vi "总磷总氮测量数据储存.vi"   [LabVIEW 2016, in "斯坦道CODcr.lvlib"]
types:
  T1 = enum16{"水样测试", "标样核查", "跨度核查", "零点核查", "加标回收", "空白测试", "平行样"}
  T2 = cluster{"时间标识":timestamp, "测量模式":enum16{"维护数据", "水样测试", "标样核查", "零点核查", "跨度核查", "空白测试", "平行样测试", "加标回收", "空白校准", "标样校准", "初始化（清洗）", "快捷测试"}, "数据标记表":string, "监测值":sgl, "单位":u16, "数据标识":string, "因子编码":u32, "标样参考值":sgl, "F0":sgl, "F1":sgl, "F2":sgl, "F3":sgl, "F4":sgl, "F5":sgl, "F6":sgl, "F7":sgl, "X":sgl, "温度":sgl, "湿度":sgl, "量程标识":string, "SN":string, "跨度值":sgl, "X1":sgl}
  T3 = enum16{"维护数据", "水样测试", "标样核查", "零点核查", "跨度核查", "空白测试", "平行样测试", "加标回收", "空白校准", "标样校准", "初始化（清洗）", "快捷测试"}
  T4 = enum16{"维护数据", "水样测试", "标样核查", "零点核查", "跨度核查", "空白测试", "平行样测试", "加标回收", "空白校准", "标样校准", "初始化（清洗）"}
  T5 = cluster{"系统时间":timestamp, "工作状态":u16, "测量模式":enum16{"待机", "连续模式", "周期模式", "定点模式", "受控模式", "手动模式"}, "告警代码":u16, "故障代码":u16, "日志代码":u16, "软件版本":u16, "F0":sgl, "F1":sgl, "F2":sgl, "F3":sgl, "T":sgl, "H":sgl, "id":u16, "flowid":u16, "量程":u16, "总磷控温温度1":sgl, "营养盐控温温度2":sgl, "ADC":sgl}
  T6 = cluster{"运行模式":enum16{"维护模式", "常规模式", "应急模式", "质控模式"}, "质控频次":enum16{"关闭", "每天", "星期一", "星期二", "星期三", "星期四", "星期五", "星期六", "星期日"}, "空白核查时间":u16, "跨度核查时间":u16, "测量间隔":u16}
  T7 = cluster{"因子编码":u32, "单位":u16, "标样参考值":sgl, "水样数据时间":timestamp, "水样实测值":sgl, "水样数据标识":string, "标样数据时间":timestamp, "标样实测值":sgl, "标样数据标识":string, "空白数据时间":timestamp, "空白实测值":sgl, "空白数据标识":string, "零点核查数据时间":timestamp, "零点核查实测值":sgl, "零点核查数据标识":string, "跨度核查数据时间":timestamp, "跨度核查实测值":sgl, "跨度核查数据标识":string, "加标回收数据时间":timestamp, "加标回收实测值":sgl, "加标回收数据标识":string, "平行样数据时间":timestamp, "平行样实测值":sgl, "平行样数据标识":string, "F0":sgl, "F1":sgl, "F2":sgl, "F3":sgl, "F4":sgl, "F5":sgl, "F6":sgl, "F7":sgl, "温度":sgl, "湿度":sgl, "X值":sgl, "fidrange":u16, "X1值":sgl}[]
  T8 = cluster{"因子编码":u32, "单位":u16, "标样参考值":sgl, "水样数据时间":timestamp, "水样实测值":sgl, "水样数据标识":string, "标样数据时间":timestamp, "标样实测值":sgl, "标样数据标识":string, "空白数据时间":timestamp, "空白实测值":sgl, "空白数据标识":string, "零点核查数据时间":timestamp, "零点核查实测值":sgl, "零点核查数据标识":string, "跨度核查数据时间":timestamp, "跨度核查实测值":sgl, "跨度核查数据标识":string, "加标回收数据时间":timestamp, "加标回收实测值":sgl, "加标回收数据标识":string, "平行样数据时间":timestamp, "平行样实测值":sgl, "平行样数据标识":string, "F0":sgl, "F1":sgl, "F2":sgl, "F3":sgl, "F4":sgl, "F5":sgl, "F6":sgl, "F7":sgl, "温度":sgl, "湿度":sgl, "X值":sgl, "fidrange":u16, "X1值":sgl}
  T9 = cluster{"总磷跨度值":dbl, "总磷零点标准液浓度":dbl, "总磷跨度标准液浓度":dbl, "总磷标准液标准浓度":dbl, "总氮跨度值":dbl, "总氮零点标准液浓度":dbl, "总氮跨度标准液浓度":dbl, "总氮标准液标准浓度":dbl, "COD跨度值":dbl, "COD零点标准液浓度":dbl, "COD跨度标准液浓度":dbl, "COD标准液标准浓度":dbl, "氨氮跨度值":dbl, "氨氮零点标准液浓度":dbl, "氨氮跨度标准液浓度":dbl, "氨氮标准液标准浓度":dbl, "磷酸盐跨度值":dbl, "磷酸盐零点标准液浓度":dbl, "磷酸盐跨度标准液浓度":dbl, "磷酸盐标准液标准浓度":dbl, "硝氮跨度值":dbl, "硝氮零点标准液浓度":dbl, "硝氮跨度标准液浓度":dbl, "硝氮标准液标准浓度":dbl, "亚硝氮跨度值":dbl, "亚硝氮零点标准液浓度":dbl, "亚硝氮跨度标准液浓度":dbl, "亚硝氮标准液标准浓度":dbl, "硫化物跨度值":dbl, "硫化物零点标准液浓度":dbl, "硫化物跨度标准液浓度":dbl, "硫化物标准液标准浓度":dbl, "硅酸盐跨度值":dbl, "硅酸盐零点标准液浓度":dbl, "硅酸盐跨度标准液浓度":dbl, "硅酸盐标准液标准浓度":dbl}
  T10 = typedef "斯坦道CODcr.lvlib/关键参数.ctl" = cluster{"测量量程":sgl, "测量检出限":sgl, "测量精度":sgl, "测量间隔":sgl, "消解温度":sgl, "消解时长":sgl, "三项式系数":sgl, "二次多项式系数":sgl, "曲线斜率":sgl, "曲线截距":sgl, "线性相关系数":sgl, "空白校准时间":timestamp, "标样校准时间":timestamp, "测量信号值":sgl, "稀释倍数":sgl, "空白标定系数":sgl, "量程系数":sgl}
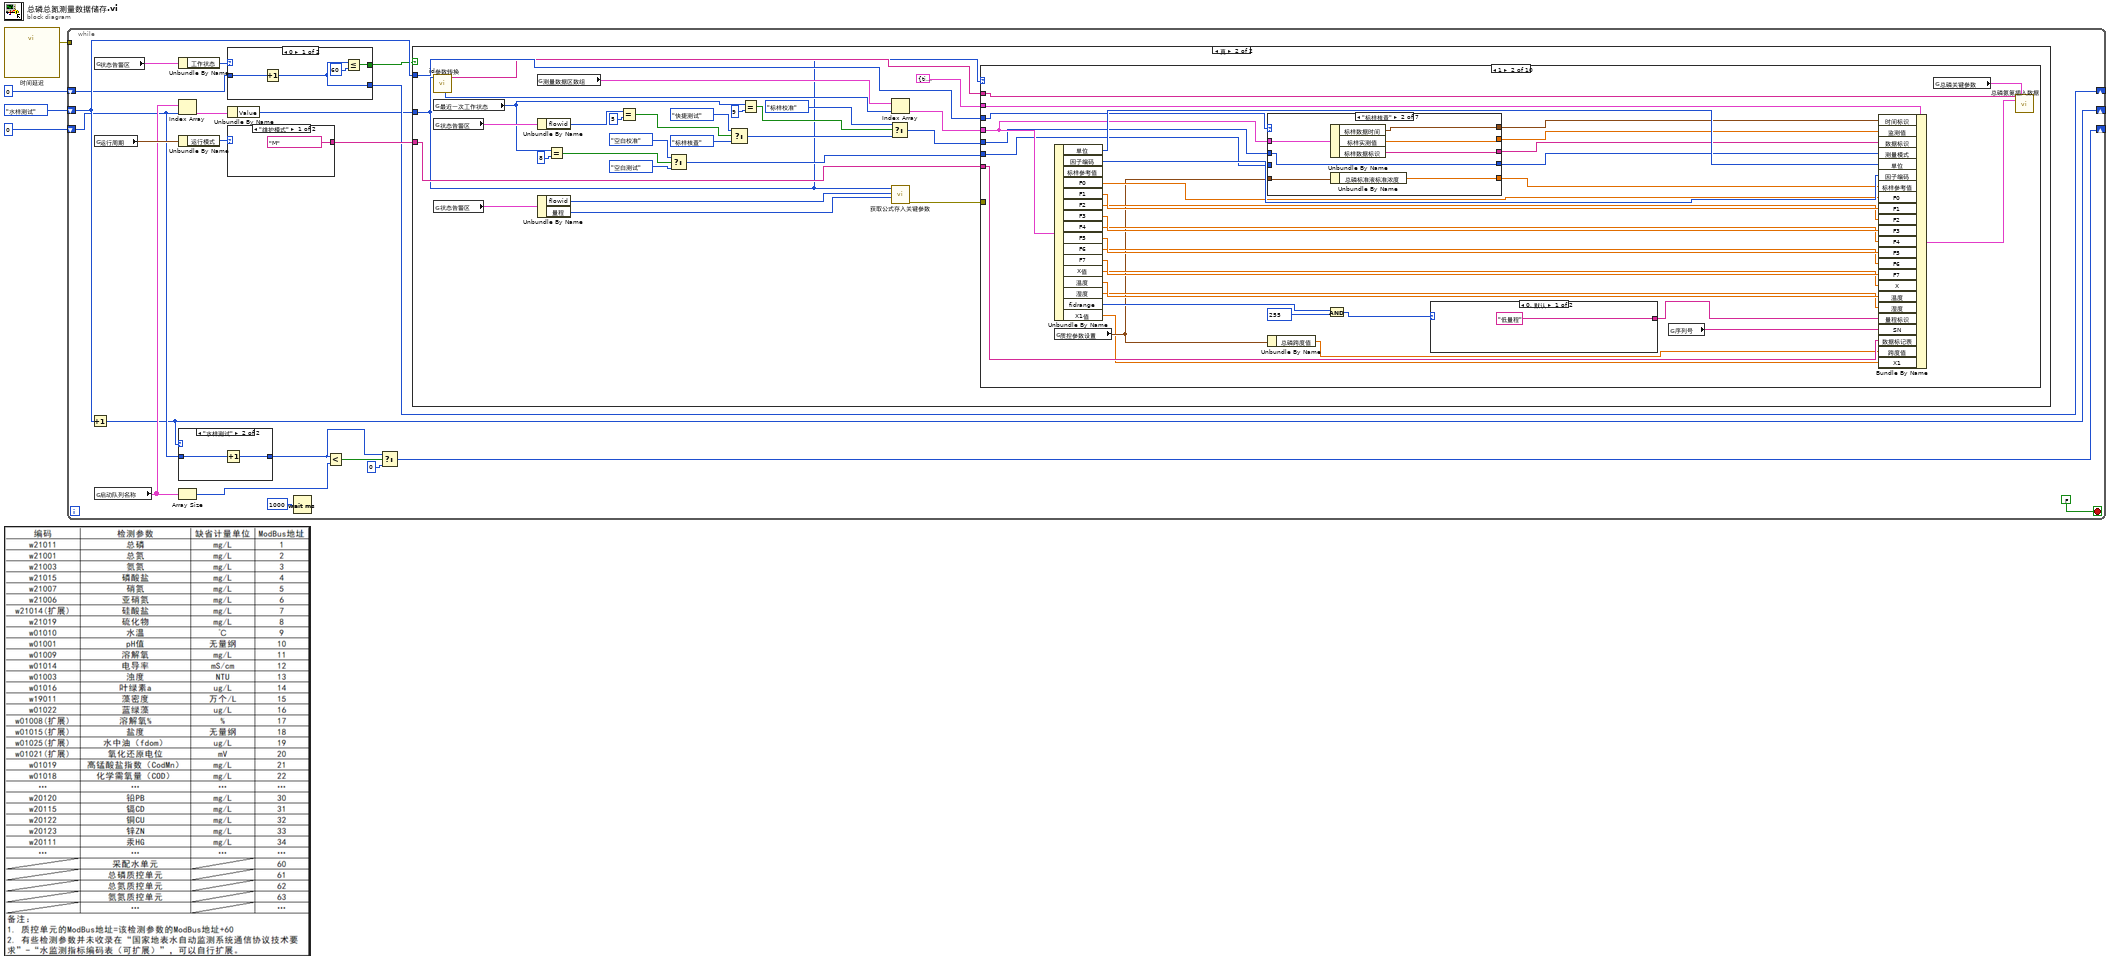
[diagram p0: block diagram]
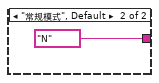
[diagram p4: hidden frame]
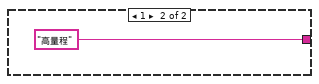
[diagram p7: hidden frame]
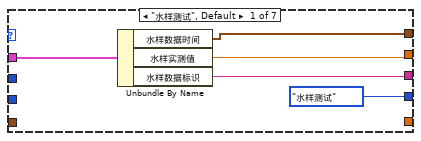
[diagram p8: hidden frame]
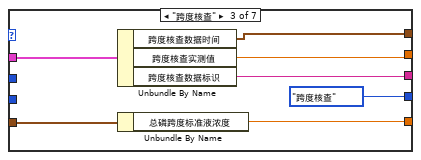
[diagram p9: hidden frame]
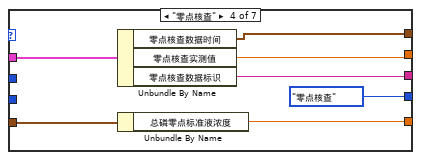
[diagram p10: hidden frame]
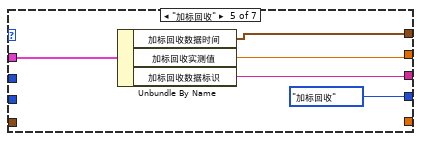
[diagram p11: hidden frame]
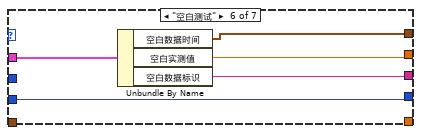
[diagram p12: hidden frame]
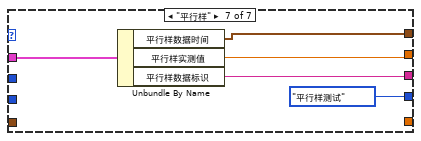
[diagram p13: hidden frame]
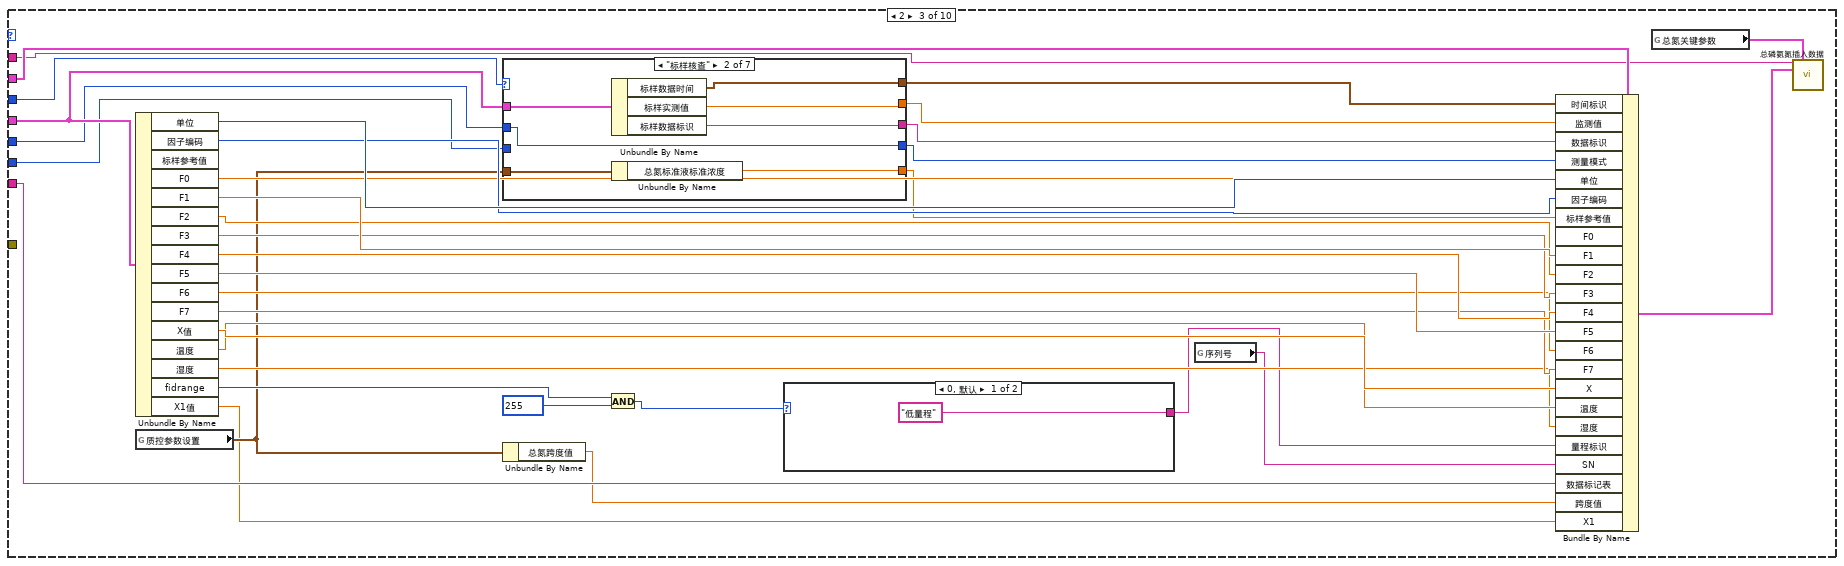
[diagram p14: hidden frame]
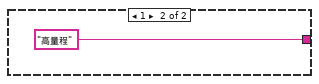
[diagram p15: hidden frame]
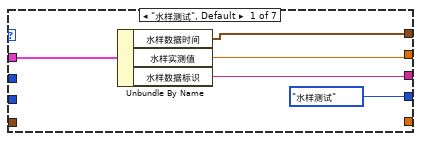
[diagram p16: hidden frame]
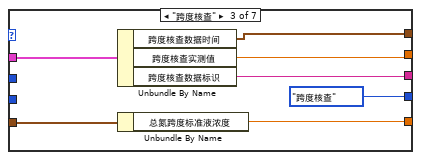
[diagram p17: hidden frame]
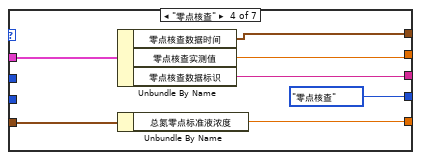
[diagram p18: hidden frame]
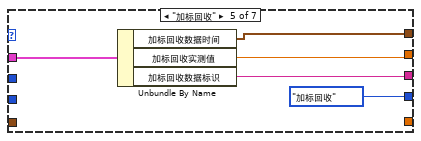
[diagram p19: hidden frame]
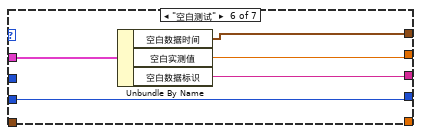
[diagram p20: hidden frame]
diagram:
  n1 = call "时间延迟"() -> ("error out"=w2:errorcluster)  [unwired: 11 in]
  n2 = while {
    shift-right: [w7] -> _
    shift-left: T1."水样测试" ("测量模式") -> [w23]
    shift-right: [w17] -> _
    shift-left: u32 0 ("等待时间（毫秒）") -> [w18]
    tunnel: w2 -> [_]
    shift-right: [w8] -> _
    shift-left: 0 -> [w11]
    stop <- FALSE stop-if-true
    n3 = Increment(x=w23) -> (x+1=w7:T1)
    n4 = global read "VAR总磷总氮全局变量.vi" "状态告警区"() -> (w20:T5)
    n5 = global read "总磷总氮断电保存全局变量.vi" "运行周期"() -> (w22:T6)
    n6 = global read "model config var.vi" "启动队列名称"() -> (w12:cluster{"String":string, "Value":u16}[])
    n7 = Unbundle By Name(w20) -> ("工作状态"=w19:u16)
    n8 = Index Array(array=w12, index=w11) -> (element=w14:cluster{"String":string, "Value":u16})
    n9 = Unbundle By Name(w22) -> ("运行模式"=w21:enum16{"维护模式", "常规模式", "应急模式", "质控模式"})
    n10 = case shown="\"水样测试\"" w7 {
      tunnel: w11 -> [w26 w28]
      tunnel: [w26 w27] -> w5
      frame Default {
      }
      frame "水样测试" {
        n11 = Increment(x=w28) -> (x+1=w27:i32)
      }
    }
    n12 = Array Size(array=w12) -> (size(s)=w10:i32)
    n13 = case shown="0" w19 {
      tunnel: w18 -> [w32 _]
      tunnel: [w31 _] -> w17
      tunnel: [w29 _] -> w16
      frame 0 {
        n14 = Increment(x=w32) -> (x+1=w31:u32)
        n15 = Less Or Equal?(x=w31, y=u32 60) -> (x <= y?=w29:bool)
      }
      frame 1, Default {
      }
    }
    n16 = Unbundle By Name(w14) -> ("Value"=w13:u16)
    n17 = case shown="\"维护模式\"" w21 {
      tunnel: ["M" ("数据标记表") "N" ("数据标记表")] -> w24
      frame "维护模式" {
      }
      frame "常规模式", Default {
      }
    }
    n18 = Wait (ms)(milliseconds to wait=u32 1000 ("等待时间（毫秒）")) -> ()  [unwired: 1 out]
    n19 = Less?(x=w5, y=w10) -> (x < y?=w9:bool)
    n20 = Select(t=w5, s=w9, f=0) -> (s? t:f=w8:i32)
    n21 = case shown="真" w16 {
      tunnel: w24 -> [_ w63]
      tunnel: w23 -> [_ w62]
      tunnel: w13 -> [_ w35]
      frame False {
      }
      frame True {
        n22 = call "id参数转换.vi"("id"=w35) -> ("table输出"=w58:string, "数组资源索引"=w57:i32)  [unwired: 9 in]
        n23 = global read "VAR总磷总氮全局变量.vi" "最近一次工作状态"() -> (w49:u16)
        n24 = global read "VAR总磷总氮全局变量.vi" "状态告警区"() -> (w61:T5)
        n25 = global read "VAR总磷总氮全局变量.vi" "状态告警区"() -> (w39:T5)
        n26 = global read "VAR总磷总氮全局变量.vi" "测量数据区数组"() -> (w60:T7)
        n27 = Unbundle By Name(w61) -> ("flowid"=w46:u16)
        n28 = Unbundle By Name(w39) -> ("flowid"=w38:u16, "量程"=w37:u16)
        n29 = Equal?(x=w49, y=u16 8) -> (x = y?=w55:bool)
        n30 = Equal?(x=w46, y=u16 5) -> (x = y?=w44:bool)
        n31 = Select(t=T3."空白校准" ("测量模式"), s=w55, f=T3."空白测试" ("测量模式")) -> (s? t:f=w48:T3)
        n32 = Select(t=T3."快捷测试" ("测量模式"), s=w44, f=T3."标样核查" ("测量模式")) -> (s? t:f=w41:T3)
        n33 = Equal?(x=w49, y=u16 9) -> (x = y?=w51:bool)
        n34 = Select(t=T3."标样校准" ("测量模式"), s=w51, f=w41) -> (s? t:f=w47:T3)
        n35 = Index Array(array=w60, index=w57) -> (element=w59:T8)
        n36 = call "获取公式存入关键参数.vi"("量程"=w37, "flowid"=w38, "id"=w35) -> ("error out"=w36:errorcluster)  [unwired: 8 in]
        n37 = case shown="1" w35 {
          tunnel: w63 -> [_ w74 w152 w231 w309 w387 w465 w543 w621 w699]
          tunnel: w62 -> [_ w82 w163 w241 w319 w397 w475 w553 w631 w709]
          tunnel: T2 {"时间标识"=timestamp(0 s since 1904-01-01), "测量模式"=enum."水样测试", "数据标记表"="N", "监测值"=0.0, "单位"=0, "数据标识"="", "因子编码"=0, "标样参考值"=0.0, "F0"=0.0, "F1"=0.0, "F2"=0.0, "F3"=0.0, "F4"=0.0, "F5"=0.0, "F6"=0.0, "F7"=0.0, "X"=0.0, "温度"=0.0, "湿度"=0.0, "量程标识"="", "SN"="", "跨度值"=0.0, "X1"=0.0} ("data") -> [_ w72 w150 w229 w307 w385 w463 w541 w619 w697]
          tunnel: w59 -> [_ w69 w147 w226 w304 w382 w460 w538 w616 w693]
          tunnel: w58 -> [_ w68 w146 w224 w302 w380 w458 w536 w614 w692]
          tunnel: w48 -> [_ w67 w145 w222 w301 w379 w457 w534 w613 w691]
          tunnel: w47 -> [_ w66 w144 w223 w300 w378 w456 w535 w612 w690]
          tunnel: w36 -> [_ _ _ _ _ _ _ _ _ _]
          frame Default {
          }
          frame 1 {
            n38 = Unbundle By Name(w69) -> ("单位"=w98:u16, "因子编码"=w97:u32, "F0"=w96:sgl, "F1"=w95:sgl, "F2"=w94:sgl, "F3"=w93:sgl, "F4"=w92:sgl, "F5"=w91:sgl, "F6"=w90:sgl, "F7"=w89:sgl, "X值"=w88:sgl, "温度"=w87:sgl, "湿度"=w86:sgl, "fidrange"=w80:u16, "X1值"=w64:sgl)  [unwired: 1 out]
            n39 = global read "总磷总氮断电保存全局变量.vi" "质控参数设置"() -> (w71:T9)
            n40 = case shown="\"标样核查\"" w82 {
              tunnel: w69 -> [w105 w112 w119 w126 w131 w136 w141]
              tunnel: [w104 w111 w118 w125 w130 w135 w140] -> w83
              tunnel: [w103 w110 w117 w124 w129 w134 w139] -> w84
              tunnel: [w102 w109 w116 w123 w128 w133 w138] -> w85
              tunnel: [T4."水样测试" ("测量模式") w106 T4."跨度核查" ("测量模式") T4."零点核查" ("测量模式") T4."加标回收" ("测量模式") w132 T4."平行样测试" ("测量模式")] -> w73
              tunnel: w71 -> [_ w108 w114 w121 _ _ _]
              tunnel: [_ w107 w113 w120 _ _ _] -> w81
              tunnel: w67 -> [_ _ _ _ _ w132 _]
              tunnel: w66 -> [_ w106 _ _ _ _ _]
              frame "水样测试", Default {
                n41 = Unbundle By Name(w105) -> ("水样数据时间"=w104:timestamp, "水样实测值"=w103:sgl, "水样数据标识"=w102:string)
              }
              frame "标样核查" {
                n42 = Unbundle By Name(w112) -> ("标样数据时间"=w111:timestamp, "标样实测值"=w110:sgl, "标样数据标识"=w109:string)
                n43 = Unbundle By Name(w108) -> ("总磷标准液标准浓度"=w107:dbl)
              }
              frame "跨度核查" {
                n44 = Unbundle By Name(w119) -> ("跨度核查数据时间"=w118:timestamp, "跨度核查实测值"=w117:sgl, "跨度核查数据标识"=w116:string)
                n45 = Unbundle By Name(w114) -> ("总磷跨度标准液浓度"=w113:dbl)
              }
              frame "零点核查" {
                n46 = Unbundle By Name(w126) -> ("零点核查数据时间"=w125:timestamp, "零点核查实测值"=w124:sgl, "零点核查数据标识"=w123:string)
                n47 = Unbundle By Name(w121) -> ("总磷零点标准液浓度"=w120:dbl)
              }
              frame "加标回收" {
                n48 = Unbundle By Name(w131) -> ("加标回收数据时间"=w130:timestamp, "加标回收实测值"=w129:sgl, "加标回收数据标识"=w128:string)
              }
              frame "空白测试" {
                n49 = Unbundle By Name(w136) -> ("空白数据时间"=w135:timestamp, "空白实测值"=w134:sgl, "空白数据标识"=w133:string)
              }
              frame "平行样" {
                n50 = Unbundle By Name(w141) -> ("平行样数据时间"=w140:timestamp, "平行样实测值"=w139:sgl, "平行样数据标识"=w138:string)
              }
            }
            n51 = Unbundle By Name(w71) -> ("总磷跨度值"=w70:dbl)
            n52 = And(x=w80, y=u16 255) -> (x .and. y?=w78:u16)
            n53 = case shown="0, 默认" w78 {
              tunnel: ["低量程" ("格式字符串") "高量程" ("格式字符串")] -> w77
              frame 0, Default {
              }
              frame 1 {
              }
            }
            n54 = global read "VAR总磷总氮全局变量.vi" "序列号"() -> (w75:string)
            n55 = Bundle By Name(cluster=w72, "时间标识"=w83, "监测值"=w84, "数据标识"=w85, "测量模式"=w73, "单位"=w98, "因子编码"=w97, "标样参考值"=w81, "F0"=w96, "F1"=w95, "F2"=w94, "F3"=w93, "F4"=w92, "F5"=w91, "F6"=w90, "F7"=w89, "X"=w88, "温度"=w87, "湿度"=w86, "量程标识"=w77, "SN"=w75, "数据标记表"=w74, "跨度值"=w70, "X1"=w64) -> (w76:T2)
            n56 = global read "VAR总磷总氮全局变量.vi" "总磷关键参数"() -> (w65:T10)
            n57 = call "总磷氨氮插入数据.vi"("table"=w68, "关键参数"=w65, "data"=w76) -> ()  [unwired: 12 in, 1 out]
          }
          frame 2 {
            n58 = Unbundle By Name(w147) -> ("单位"=w176:u16, "因子编码"=w175:u32, "F0"=w174:sgl, "F1"=w173:sgl, "F2"=w172:sgl, "F3"=w171:sgl, "F4"=w170:sgl, "F5"=w169:sgl, "F6"=w168:sgl, "F7"=w167:sgl, "X值"=w166:sgl, "温度"=w165:sgl, "湿度"=w164:sgl, "fidrange"=w156:u16, "X1值"=w142:sgl)  [unwired: 1 out]
            n59 = global read "总磷总氮断电保存全局变量.vi" "质控参数设置"() -> (w149:T9)
            n60 = case shown="\"标样核查\"" w163 {
              tunnel: w147 -> [w183 w190 w197 w204 w209 w214 w219]
              tunnel: [w182 w189 w196 w203 w208 w213 w218] -> w162
              tunnel: [w181 w188 w195 w202 w207 w212 w217] -> w161
              tunnel: [w180 w187 w194 w201 w206 w211 w216] -> w160
              tunnel: [T4."水样测试" ("测量模式") w184 T4."跨度核查" ("测量模式") T4."零点核查" ("测量模式") T4."加标回收" ("测量模式") w210 T4."平行样测试" ("测量模式")] -> w151
              tunnel: w149 -> [_ w186 w192 w199 _ _ _]
              tunnel: [_ w185 w191 w198 _ _ _] -> w159
              tunnel: w145 -> [_ _ _ _ _ w210 _]
              tunnel: w144 -> [_ w184 _ _ _ _ _]
              frame "水样测试", Default {
                n61 = Unbundle By Name(w183) -> ("水样数据时间"=w182:timestamp, "水样实测值"=w181:sgl, "水样数据标识"=w180:string)
              }
              frame "标样核查" {
                n62 = Unbundle By Name(w190) -> ("标样数据时间"=w189:timestamp, "标样实测值"=w188:sgl, "标样数据标识"=w187:string)
                n63 = Unbundle By Name(w186) -> ("总氮标准液标准浓度"=w185:dbl)
              }
              frame "跨度核查" {
                n64 = Unbundle By Name(w197) -> ("跨度核查数据时间"=w196:timestamp, "跨度核查实测值"=w195:sgl, "跨度核查数据标识"=w194:string)
                n65 = Unbundle By Name(w192) -> ("总氮跨度标准液浓度"=w191:dbl)
              }
              frame "零点核查" {
                n66 = Unbundle By Name(w204) -> ("零点核查数据时间"=w203:timestamp, "零点核查实测值"=w202:sgl, "零点核查数据标识"=w201:string)
                n67 = Unbundle By Name(w199) -> ("总氮零点标准液浓度"=w198:dbl)
              }
              frame "加标回收" {
                n68 = Unbundle By Name(w209) -> ("加标回收数据时间"=w208:timestamp, "加标回收实测值"=w207:sgl, "加标回收数据标识"=w206:string)
              }
              frame "空白测试" {
                n69 = Unbundle By Name(w214) -> ("空白数据时间"=w213:timestamp, "空白实测值"=w212:sgl, "空白数据标识"=w211:string)
              }
              frame "平行样" {
                n70 = Unbundle By Name(w219) -> ("平行样数据时间"=w218:timestamp, "平行样实测值"=w217:sgl, "平行样数据标识"=w216:string)
              }
            }
            n71 = Unbundle By Name(w149) -> ("总氮跨度值"=w148:dbl)
            n72 = And(x=w156, y=u16 255) -> (x .and. y?=w157:u16)
            n73 = case shown="0, 默认" w157 {
              tunnel: ["低量程" ("格式字符串") "高量程" ("格式字符串")] -> w155
              frame 0, Default {
              }
              frame 1 {
              }
            }
            n74 = global read "VAR总磷总氮全局变量.vi" "序列号"() -> (w153:string)
            n75 = Bundle By Name(cluster=w150, "时间标识"=w162, "监测值"=w161, "数据标识"=w160, "测量模式"=w151, "单位"=w176, "因子编码"=w175, "标样参考值"=w159, "F0"=w174, "F1"=w173, "F2"=w172, "F3"=w171, "F4"=w170, "F5"=w169, "F6"=w168, "F7"=w167, "X"=w166, "温度"=w165, "湿度"=w164, "量程标识"=w155, "SN"=w153, "数据标记表"=w152, "跨度值"=w148, "X1"=w142) -> (w154:T2)
            n76 = global read "VAR总磷总氮全局变量.vi" "总氮关键参数"() -> (w143:T10)
            n77 = call "总磷氨氮插入数据.vi"("table"=w146, "关键参数"=w143, "data"=w154) -> ()  [unwired: 12 in, 1 out]
          }
          frame 3 {
            n78 = Unbundle By Name(w226) -> ("单位"=w254:u16, "因子编码"=w253:u32, "F0"=w252:sgl, "F1"=w251:sgl, "F2"=w250:sgl, "F3"=w249:sgl, "F4"=w248:sgl, "F5"=w247:sgl, "F6"=w246:sgl, "F7"=w245:sgl, "X值"=w244:sgl, "温度"=w243:sgl, "湿度"=w242:sgl, "fidrange"=w234:u16, "X1值"=w220:sgl)  [unwired: 1 out]
            n79 = global read "总磷总氮断电保存全局变量.vi" "质控参数设置"() -> (w228:T9)
            n80 = case shown="\"空白测试\"" w241 {
              tunnel: w226 -> [w261 w268 w275 w282 w287 w292 w297]
              tunnel: [w260 w267 w274 w281 w286 w291 w296] -> w240
              tunnel: [w259 w266 w273 w280 w285 w290 w295] -> w239
              tunnel: [w258 w265 w272 w279 w284 w289 w294] -> w238
              tunnel: [T4."水样测试" ("测量模式") w262 T4."跨度核查" ("测量模式") T4."零点核查" ("测量模式") T4."加标回收" ("测量模式") w288 T4."平行样测试" ("测量模式")] -> w230
              tunnel: w228 -> [_ w264 w270 w277 _ _ _]
              tunnel: [_ w263 w269 w276 _ _ _] -> w237
              tunnel: w223 -> [_ w262 _ _ _ _ _]
              tunnel: w222 -> [_ _ _ _ _ w288 _]
              frame "水样测试", Default {
                n81 = Unbundle By Name(w261) -> ("水样数据时间"=w260:timestamp, "水样实测值"=w259:sgl, "水样数据标识"=w258:string)
              }
              frame "标样核查" {
                n82 = Unbundle By Name(w268) -> ("标样数据时间"=w267:timestamp, "标样实测值"=w266:sgl, "标样数据标识"=w265:string)
                n83 = Unbundle By Name(w264) -> ("氨氮标准液标准浓度"=w263:dbl)
              }
              frame "跨度核查" {
                n84 = Unbundle By Name(w275) -> ("跨度核查数据时间"=w274:timestamp, "跨度核查实测值"=w273:sgl, "跨度核查数据标识"=w272:string)
                n85 = Unbundle By Name(w270) -> ("氨氮跨度标准液浓度"=w269:dbl)
              }
              frame "零点核查" {
                n86 = Unbundle By Name(w282) -> ("零点核查数据时间"=w281:timestamp, "零点核查实测值"=w280:sgl, "零点核查数据标识"=w279:string)
                n87 = Unbundle By Name(w277) -> ("氨氮零点标准液浓度"=w276:dbl)
              }
              frame "加标回收" {
                n88 = Unbundle By Name(w287) -> ("加标回收数据时间"=w286:timestamp, "加标回收实测值"=w285:sgl, "加标回收数据标识"=w284:string)
              }
              frame "空白测试" {
                n89 = Unbundle By Name(w292) -> ("空白数据时间"=w291:timestamp, "空白实测值"=w290:sgl, "空白数据标识"=w289:string)
              }
              frame "平行样" {
                n90 = Unbundle By Name(w297) -> ("平行样数据时间"=w296:timestamp, "平行样实测值"=w295:sgl, "平行样数据标识"=w294:string)
              }
            }
            n91 = Unbundle By Name(w228) -> ("氨氮跨度值"=w227:dbl)
            n92 = And(x=w234, y=u16 255) -> (x .and. y?=w235:u16)
            n93 = case shown="0, 默认" w235 {
              tunnel: ["低量程" ("格式字符串") "高量程" ("格式字符串")] -> w233
              frame 0, Default {
              }
              frame 1 {
              }
            }
            n94 = global read "VAR总磷总氮全局变量.vi" "序列号"() -> (w232:string)
            n95 = Bundle By Name(cluster=w229, "时间标识"=w240, "监测值"=w239, "数据标识"=w238, "测量模式"=w230, "单位"=w254, "因子编码"=w253, "标样参考值"=w237, "F0"=w252, "F1"=w251, "F2"=w250, "F3"=w249, "F4"=w248, "F5"=w247, "F6"=w246, "F7"=w245, "X"=w244, "温度"=w243, "湿度"=w242, "量程标识"=w233, "SN"=w232, "数据标记表"=w231, "跨度值"=w227, "X1"=w220) -> (w225:T2)
            n96 = global read "VAR总磷总氮全局变量.vi" "氨氮关键参数"() -> (w221:T10)
            n97 = call "总磷氨氮插入数据.vi"("table"=w224, "关键参数"=w221, "data"=w225) -> ()  [unwired: 12 in, 1 out]
          }
          frame 4 {
            n98 = Unbundle By Name(w304) -> ("单位"=w332:u16, "因子编码"=w331:u32, "F0"=w330:sgl, "F1"=w329:sgl, "F2"=w328:sgl, "F3"=w327:sgl, "F4"=w326:sgl, "F5"=w325:sgl, "F6"=w324:sgl, "F7"=w323:sgl, "X值"=w322:sgl, "温度"=w321:sgl, "湿度"=w320:sgl, "fidrange"=w312:u16, "X1值"=w298:sgl)  [unwired: 1 out]
            n99 = global read "总磷总氮断电保存全局变量.vi" "质控参数设置"() -> (w306:T9)
            n100 = case shown="\"标样核查\"" w319 {
              tunnel: w304 -> [w339 w346 w353 w360 w365 w370 w375]
              tunnel: [w338 w345 w352 w359 w364 w369 w374] -> w318
              tunnel: [w337 w344 w351 w358 w363 w368 w373] -> w317
              tunnel: [w336 w343 w350 w357 w362 w367 w372] -> w316
              tunnel: [T4."水样测试" ("测量模式") w340 T4."跨度核查" ("测量模式") T4."零点核查" ("测量模式") T4."加标回收" ("测量模式") w366 T4."平行样测试" ("测量模式")] -> w308
              tunnel: w306 -> [_ w342 w348 w355 _ _ _]
              tunnel: [_ w341 w347 w354 _ _ _] -> w315
              tunnel: w301 -> [_ _ _ _ _ w366 _]
              tunnel: w300 -> [_ w340 _ _ _ _ _]
              frame "水样测试", Default {
                n101 = Unbundle By Name(w339) -> ("水样数据时间"=w338:timestamp, "水样实测值"=w337:sgl, "水样数据标识"=w336:string)
              }
              frame "标样核查" {
                n102 = Unbundle By Name(w346) -> ("标样数据时间"=w345:timestamp, "标样实测值"=w344:sgl, "标样数据标识"=w343:string)
                n103 = Unbundle By Name(w342) -> ("磷酸盐标准液标准浓度"=w341:dbl)
              }
              frame "跨度核查" {
                n104 = Unbundle By Name(w353) -> ("跨度核查数据时间"=w352:timestamp, "跨度核查实测值"=w351:sgl, "跨度核查数据标识"=w350:string)
                n105 = Unbundle By Name(w348) -> ("磷酸盐跨度标准液浓度"=w347:dbl)
              }
              frame "零点核查" {
                n106 = Unbundle By Name(w360) -> ("零点核查数据时间"=w359:timestamp, "零点核查实测值"=w358:sgl, "零点核查数据标识"=w357:string)
                n107 = Unbundle By Name(w355) -> ("磷酸盐零点标准液浓度"=w354:dbl)
              }
              frame "加标回收" {
                n108 = Unbundle By Name(w365) -> ("加标回收数据时间"=w364:timestamp, "加标回收实测值"=w363:sgl, "加标回收数据标识"=w362:string)
              }
              frame "空白测试" {
                n109 = Unbundle By Name(w370) -> ("空白数据时间"=w369:timestamp, "空白实测值"=w368:sgl, "空白数据标识"=w367:string)
              }
              frame "平行样" {
                n110 = Unbundle By Name(w375) -> ("平行样数据时间"=w374:timestamp, "平行样实测值"=w373:sgl, "平行样数据标识"=w372:string)
              }
            }
            n111 = Unbundle By Name(w306) -> ("磷酸盐跨度值"=w305:dbl)
            n112 = And(x=w312, y=u16 255) -> (x .and. y?=w313:u16)
            n113 = case shown="0, 默认" w313 {
              tunnel: ["低量程" ("格式字符串") "高量程" ("格式字符串")] -> w311
              frame 0, Default {
              }
              frame 1 {
              }
            }
            n114 = global read "VAR总磷总氮全局变量.vi" "序列号"() -> (w310:string)
            n115 = Bundle By Name(cluster=w307, "时间标识"=w318, "监测值"=w317, "数据标识"=w316, "测量模式"=w308, "单位"=w332, "因子编码"=w331, "标样参考值"=w315, "F0"=w330, "F1"=w329, "F2"=w328, "F3"=w327, "F4"=w326, "F5"=w325, "F6"=w324, "F7"=w323, "X"=w322, "温度"=w321, "湿度"=w320, "量程标识"=w311, "SN"=w310, "数据标记表"=w309, "跨度值"=w305, "X1"=w298) -> (w303:T2)
            n116 = global read "VAR总磷总氮全局变量.vi" "磷酸盐关键参数"() -> (w299:T10)
            n117 = call "总磷氨氮插入数据.vi"("table"=w302, "关键参数"=w299, "data"=w303) -> ()  [unwired: 12 in, 1 out]
          }
          frame 5 {
            n118 = Unbundle By Name(w382) -> ("单位"=w410:u16, "因子编码"=w409:u32, "F0"=w408:sgl, "F1"=w407:sgl, "F2"=w406:sgl, "F3"=w405:sgl, "F4"=w404:sgl, "F5"=w403:sgl, "F6"=w402:sgl, "F7"=w401:sgl, "X值"=w400:sgl, "温度"=w399:sgl, "湿度"=w398:sgl, "fidrange"=w390:u16, "X1值"=w376:sgl)  [unwired: 1 out]
            n119 = global read "总磷总氮断电保存全局变量.vi" "质控参数设置"() -> (w384:T9)
            n120 = case shown="\"标样核查\"" w397 {
              tunnel: w382 -> [w417 w424 w431 w438 w443 w448 w453]
              tunnel: [w416 w423 w430 w437 w442 w447 w452] -> w396
              tunnel: [w415 w422 w429 w436 w441 w446 w451] -> w395
              tunnel: [w414 w421 w428 w435 w440 w445 w450] -> w394
              tunnel: [T4."水样测试" ("测量模式") w418 T4."跨度核查" ("测量模式") T4."零点核查" ("测量模式") T4."加标回收" ("测量模式") w444 T4."平行样测试" ("测量模式")] -> w386
              tunnel: w384 -> [_ w420 w426 w433 _ _ _]
              tunnel: [_ w419 w425 w432 _ _ _] -> w393
              tunnel: w379 -> [_ _ _ _ _ w444 _]
              tunnel: w378 -> [_ w418 _ _ _ _ _]
              frame "水样测试", Default {
                n121 = Unbundle By Name(w417) -> ("水样数据时间"=w416:timestamp, "水样实测值"=w415:sgl, "水样数据标识"=w414:string)
              }
              frame "标样核查" {
                n122 = Unbundle By Name(w424) -> ("标样数据时间"=w423:timestamp, "标样实测值"=w422:sgl, "标样数据标识"=w421:string)
                n123 = Unbundle By Name(w420) -> ("硝氮标准液标准浓度"=w419:dbl)
              }
              frame "跨度核查" {
                n124 = Unbundle By Name(w431) -> ("跨度核查数据时间"=w430:timestamp, "跨度核查实测值"=w429:sgl, "跨度核查数据标识"=w428:string)
                n125 = Unbundle By Name(w426) -> ("硝氮跨度标准液浓度"=w425:dbl)
              }
              frame "零点核查" {
                n126 = Unbundle By Name(w438) -> ("零点核查数据时间"=w437:timestamp, "零点核查实测值"=w436:sgl, "零点核查数据标识"=w435:string)
                n127 = Unbundle By Name(w433) -> ("硝氮零点标准液浓度"=w432:dbl)
              }
              frame "加标回收" {
                n128 = Unbundle By Name(w443) -> ("加标回收数据时间"=w442:timestamp, "加标回收实测值"=w441:sgl, "加标回收数据标识"=w440:string)
              }
              frame "空白测试" {
                n129 = Unbundle By Name(w448) -> ("空白数据时间"=w447:timestamp, "空白实测值"=w446:sgl, "空白数据标识"=w445:string)
              }
              frame "平行样" {
                n130 = Unbundle By Name(w453) -> ("平行样数据时间"=w452:timestamp, "平行样实测值"=w451:sgl, "平行样数据标识"=w450:string)
              }
            }
            n131 = Unbundle By Name(w384) -> ("硝氮跨度值"=w383:dbl)
            n132 = And(x=w390, y=u16 255) -> (x .and. y?=w391:u16)
            n133 = case shown="0, 默认" w391 {
              tunnel: ["低量程" ("格式字符串") "高量程" ("格式字符串")] -> w389
              frame 0, Default {
              }
              frame 1 {
              }
            }
            n134 = global read "VAR总磷总氮全局变量.vi" "序列号"() -> (w388:string)
            n135 = Bundle By Name(cluster=w385, "时间标识"=w396, "监测值"=w395, "数据标识"=w394, "测量模式"=w386, "单位"=w410, "因子编码"=w409, "标样参考值"=w393, "F0"=w408, "F1"=w407, "F2"=w406, "F3"=w405, "F4"=w404, "F5"=w403, "F6"=w402, "F7"=w401, "X"=w400, "温度"=w399, "湿度"=w398, "量程标识"=w389, "SN"=w388, "数据标记表"=w387, "跨度值"=w383, "X1"=w376) -> (w381:T2)
            n136 = global read "VAR总磷总氮全局变量.vi" "硝氮关键参数"() -> (w377:T10)
            n137 = call "总磷氨氮插入数据.vi"("table"=w380, "关键参数"=w377, "data"=w381) -> ()  [unwired: 12 in, 1 out]
          }
          frame 6 {
            n138 = Unbundle By Name(w460) -> ("单位"=w488:u16, "因子编码"=w487:u32, "F0"=w486:sgl, "F1"=w485:sgl, "F2"=w484:sgl, "F3"=w483:sgl, "F4"=w482:sgl, "F5"=w481:sgl, "F6"=w480:sgl, "F7"=w479:sgl, "X值"=w478:sgl, "温度"=w477:sgl, "湿度"=w476:sgl, "fidrange"=w468:u16, "X1值"=w454:sgl)  [unwired: 1 out]
            n139 = global read "总磷总氮断电保存全局变量.vi" "质控参数设置"() -> (w462:T9)
            n140 = case shown="\"标样核查\"" w475 {
              tunnel: w460 -> [w495 w502 w509 w516 w521 w526 w531]
              tunnel: [w494 w501 w508 w515 w520 w525 w530] -> w474
              tunnel: [w493 w500 w507 w514 w519 w524 w529] -> w473
              tunnel: [w492 w499 w506 w513 w518 w523 w528] -> w472
              tunnel: [T4."水样测试" ("测量模式") w496 T4."跨度核查" ("测量模式") T4."零点核查" ("测量模式") T4."加标回收" ("测量模式") w522 T4."平行样测试" ("测量模式")] -> w464
              tunnel: w462 -> [_ w498 w504 w511 _ _ _]
              tunnel: [_ w497 w503 w510 _ _ _] -> w471
              tunnel: w457 -> [_ _ _ _ _ w522 _]
              tunnel: w456 -> [_ w496 _ _ _ _ _]
              frame "水样测试", Default {
                n141 = Unbundle By Name(w495) -> ("水样数据时间"=w494:timestamp, "水样实测值"=w493:sgl, "水样数据标识"=w492:string)
              }
              frame "标样核查" {
                n142 = Unbundle By Name(w502) -> ("标样数据时间"=w501:timestamp, "标样实测值"=w500:sgl, "标样数据标识"=w499:string)
                n143 = Unbundle By Name(w498) -> ("亚硝氮标准液标准浓度"=w497:dbl)
              }
              frame "跨度核查" {
                n144 = Unbundle By Name(w509) -> ("跨度核查数据时间"=w508:timestamp, "跨度核查实测值"=w507:sgl, "跨度核查数据标识"=w506:string)
                n145 = Unbundle By Name(w504) -> ("亚硝氮跨度标准液浓度"=w503:dbl)
              }
              frame "零点核查" {
                n146 = Unbundle By Name(w516) -> ("零点核查数据时间"=w515:timestamp, "零点核查实测值"=w514:sgl, "零点核查数据标识"=w513:string)
                n147 = Unbundle By Name(w511) -> ("亚硝氮零点标准液浓度"=w510:dbl)
              }
              frame "加标回收" {
                n148 = Unbundle By Name(w521) -> ("加标回收数据时间"=w520:timestamp, "加标回收实测值"=w519:sgl, "加标回收数据标识"=w518:string)
              }
              frame "空白测试" {
                n149 = Unbundle By Name(w526) -> ("空白数据时间"=w525:timestamp, "空白实测值"=w524:sgl, "空白数据标识"=w523:string)
              }
              frame "平行样" {
                n150 = Unbundle By Name(w531) -> ("平行样数据时间"=w530:timestamp, "平行样实测值"=w529:sgl, "平行样数据标识"=w528:string)
              }
            }
            n151 = Unbundle By Name(w462) -> ("亚硝氮跨度值"=w461:dbl)
            n152 = And(x=w468, y=u16 255) -> (x .and. y?=w469:u16)
            n153 = case shown="0, 默认" w469 {
              tunnel: ["低量程" ("格式字符串") "高量程" ("格式字符串")] -> w467
              frame 0, Default {
              }
              frame 1 {
              }
            }
            n154 = global read "VAR总磷总氮全局变量.vi" "序列号"() -> (w466:string)
            n155 = Bundle By Name(cluster=w463, "时间标识"=w474, "监测值"=w473, "数据标识"=w472, "测量模式"=w464, "单位"=w488, "因子编码"=w487, "标样参考值"=w471, "F0"=w486, "F1"=w485, "F2"=w484, "F3"=w483, "F4"=w482, "F5"=w481, "F6"=w480, "F7"=w479, "X"=w478, "温度"=w477, "湿度"=w476, "量程标识"=w467, "SN"=w466, "数据标记表"=w465, "跨度值"=w461, "X1"=w454) -> (w459:T2)
            n156 = global read "VAR总磷总氮全局变量.vi" "亚硝氮关键参数"() -> (w455:T10)
            n157 = call "总磷氨氮插入数据.vi"("table"=w458, "关键参数"=w455, "data"=w459) -> ()  [unwired: 12 in, 1 out]
          }
          frame 7 {
            n158 = Unbundle By Name(w538) -> ("单位"=w566:u16, "因子编码"=w565:u32, "F0"=w564:sgl, "F1"=w563:sgl, "F2"=w562:sgl, "F3"=w561:sgl, "F4"=w560:sgl, "F5"=w559:sgl, "F6"=w558:sgl, "F7"=w557:sgl, "X值"=w556:sgl, "温度"=w555:sgl, "湿度"=w554:sgl, "fidrange"=w546:u16, "X1值"=w532:sgl)  [unwired: 1 out]
            n159 = global read "总磷总氮断电保存全局变量.vi" "质控参数设置"() -> (w540:T9)
            n160 = case shown="\"空白测试\"" w553 {
              tunnel: w538 -> [w573 w580 w587 w594 w599 w604 w609]
              tunnel: [w572 w579 w586 w593 w598 w603 w608] -> w552
              tunnel: [w571 w578 w585 w592 w597 w602 w607] -> w551
              tunnel: [w570 w577 w584 w591 w596 w601 w606] -> w550
              tunnel: [T4."水样测试" ("测量模式") w574 T4."跨度核查" ("测量模式") T4."零点核查" ("测量模式") T4."加标回收" ("测量模式") w600 T4."平行样测试" ("测量模式")] -> w542
              tunnel: w540 -> [_ w576 w582 w589 _ _ _]
              tunnel: [_ w575 w581 w588 _ _ _] -> w549
              tunnel: w535 -> [_ w574 _ _ _ _ _]
              tunnel: w534 -> [_ _ _ _ _ w600 _]
              frame "水样测试", Default {
                n161 = Unbundle By Name(w573) -> ("水样数据时间"=w572:timestamp, "水样实测值"=w571:sgl, "水样数据标识"=w570:string)
              }
              frame "标样核查" {
                n162 = Unbundle By Name(w580) -> ("标样数据时间"=w579:timestamp, "标样实测值"=w578:sgl, "标样数据标识"=w577:string)
                n163 = Unbundle By Name(w576) -> ("硅酸盐标准液标准浓度"=w575:dbl)
              }
              frame "跨度核查" {
                n164 = Unbundle By Name(w587) -> ("跨度核查数据时间"=w586:timestamp, "跨度核查实测值"=w585:sgl, "跨度核查数据标识"=w584:string)
                n165 = Unbundle By Name(w582) -> ("硅酸盐跨度标准液浓度"=w581:dbl)
              }
              frame "零点核查" {
                n166 = Unbundle By Name(w594) -> ("零点核查数据时间"=w593:timestamp, "零点核查实测值"=w592:sgl, "零点核查数据标识"=w591:string)
                n167 = Unbundle By Name(w589) -> ("硅酸盐零点标准液浓度"=w588:dbl)
              }
              frame "加标回收" {
                n168 = Unbundle By Name(w599) -> ("加标回收数据时间"=w598:timestamp, "加标回收实测值"=w597:sgl, "加标回收数据标识"=w596:string)
              }
              frame "空白测试" {
                n169 = Unbundle By Name(w604) -> ("空白数据时间"=w603:timestamp, "空白实测值"=w602:sgl, "空白数据标识"=w601:string)
              }
              frame "平行样" {
                n170 = Unbundle By Name(w609) -> ("平行样数据时间"=w608:timestamp, "平行样实测值"=w607:sgl, "平行样数据标识"=w606:string)
              }
            }
            n171 = Unbundle By Name(w540) -> ("硅酸盐跨度值"=w539:dbl)
            n172 = And(x=w546, y=u16 255) -> (x .and. y?=w547:u16)
            n173 = case shown="0, 默认" w547 {
              tunnel: ["低量程" ("格式字符串") "高量程" ("格式字符串")] -> w545
              frame 0, Default {
              }
              frame 1 {
              }
            }
            n174 = global read "VAR总磷总氮全局变量.vi" "序列号"() -> (w544:string)
            n175 = Bundle By Name(cluster=w541, "时间标识"=w552, "监测值"=w551, "数据标识"=w550, "测量模式"=w542, "单位"=w566, "因子编码"=w565, "标样参考值"=w549, "F0"=w564, "F1"=w563, "F2"=w562, "F3"=w561, "F4"=w560, "F5"=w559, "F6"=w558, "F7"=w557, "X"=w556, "温度"=w555, "湿度"=w554, "量程标识"=w545, "SN"=w544, "数据标记表"=w543, "跨度值"=w539, "X1"=w532) -> (w537:T2)
            n176 = global read "VAR总磷总氮全局变量.vi" "硅酸盐关键参数"() -> (w533:T10)
            n177 = call "总磷氨氮插入数据.vi"("table"=w536, "关键参数"=w533, "data"=w537) -> ()  [unwired: 12 in, 1 out]
          }
          frame 8 {
            n178 = Unbundle By Name(w616) -> ("单位"=w644:u16, "因子编码"=w643:u32, "F0"=w642:sgl, "F1"=w641:sgl, "F2"=w640:sgl, "F3"=w639:sgl, "F4"=w638:sgl, "F5"=w637:sgl, "F6"=w636:sgl, "F7"=w635:sgl, "X值"=w634:sgl, "温度"=w633:sgl, "湿度"=w632:sgl, "fidrange"=w624:u16, "X1值"=w610:sgl)  [unwired: 1 out]
            n179 = global read "总磷总氮断电保存全局变量.vi" "质控参数设置"() -> (w618:T9)
            n180 = case shown="\"标样核查\"" w631 {
              tunnel: w616 -> [w651 w658 w665 w672 w677 w682 w687]
              tunnel: [w650 w657 w664 w671 w676 w681 w686] -> w630
              tunnel: [w649 w656 w663 w670 w675 w680 w685] -> w629
              tunnel: [w648 w655 w662 w669 w674 w679 w684] -> w628
              tunnel: [T4."水样测试" ("测量模式") w652 T4."跨度核查" ("测量模式") T4."零点核查" ("测量模式") T4."加标回收" ("测量模式") w678 T4."平行样测试" ("测量模式")] -> w620
              tunnel: w618 -> [_ w654 w660 w667 _ _ _]
              tunnel: [_ w653 w659 w666 _ _ _] -> w627
              tunnel: w613 -> [_ _ _ _ _ w678 _]
              tunnel: w612 -> [_ w652 _ _ _ _ _]
              frame "水样测试", Default {
                n181 = Unbundle By Name(w651) -> ("水样数据时间"=w650:timestamp, "水样实测值"=w649:sgl, "水样数据标识"=w648:string)
              }
              frame "标样核查" {
                n182 = Unbundle By Name(w658) -> ("标样数据时间"=w657:timestamp, "标样实测值"=w656:sgl, "标样数据标识"=w655:string)
                n183 = Unbundle By Name(w654) -> ("硫化物标准液标准浓度"=w653:dbl)
              }
              frame "跨度核查" {
                n184 = Unbundle By Name(w665) -> ("跨度核查数据时间"=w664:timestamp, "跨度核查实测值"=w663:sgl, "跨度核查数据标识"=w662:string)
                n185 = Unbundle By Name(w660) -> ("硫化物跨度标准液浓度"=w659:dbl)
              }
              frame "零点核查" {
                n186 = Unbundle By Name(w672) -> ("零点核查数据时间"=w671:timestamp, "零点核查实测值"=w670:sgl, "零点核查数据标识"=w669:string)
                n187 = Unbundle By Name(w667) -> ("硫化物零点标准液浓度"=w666:dbl)
              }
              frame "加标回收" {
                n188 = Unbundle By Name(w677) -> ("加标回收数据时间"=w676:timestamp, "加标回收实测值"=w675:sgl, "加标回收数据标识"=w674:string)
              }
              frame "空白测试" {
                n189 = Unbundle By Name(w682) -> ("空白数据时间"=w681:timestamp, "空白实测值"=w680:sgl, "空白数据标识"=w679:string)
              }
              frame "平行样" {
                n190 = Unbundle By Name(w687) -> ("平行样数据时间"=w686:timestamp, "平行样实测值"=w685:sgl, "平行样数据标识"=w684:string)
              }
            }
            n191 = Unbundle By Name(w618) -> ("硫化物跨度值"=w617:dbl)
            n192 = And(x=w624, y=u16 255) -> (x .and. y?=w625:u16)
            n193 = case shown="0, 默认" w625 {
              tunnel: ["低量程" ("格式字符串") "高量程" ("格式字符串")] -> w623
              frame 0, Default {
              }
              frame 1 {
              }
            }
            n194 = global read "VAR总磷总氮全局变量.vi" "序列号"() -> (w622:string)
            n195 = Bundle By Name(cluster=w619, "时间标识"=w630, "监测值"=w629, "数据标识"=w628, "测量模式"=w620, "单位"=w644, "因子编码"=w643, "标样参考值"=w627, "F0"=w642, "F1"=w641, "F2"=w640, "F3"=w639, "F4"=w638, "F5"=w637, "F6"=w636, "F7"=w635, "X"=w634, "温度"=w633, "湿度"=w632, "量程标识"=w623, "SN"=w622, "数据标记表"=w621, "跨度值"=w617, "X1"=w610) -> (w615:T2)
            n196 = global read "VAR总磷总氮全局变量.vi" "硫化物关键参数"() -> (w611:T10)
            n197 = call "总磷氨氮插入数据.vi"("table"=w614, "关键参数"=w611, "data"=w615) -> ()  [unwired: 12 in, 1 out]
          }
          frame 22 {
            n198 = Unbundle By Name(w693) -> ("单位"=w722:u16, "因子编码"=w721:u32, "F0"=w720:sgl, "F1"=w719:sgl, "F2"=w718:sgl, "F3"=w717:sgl, "F4"=w716:sgl, "F5"=w715:sgl, "F6"=w714:sgl, "F7"=w713:sgl, "X值"=w712:sgl, "温度"=w711:sgl, "湿度"=w710:sgl, "fidrange"=w702:u16, "X1值"=w688:sgl)  [unwired: 1 out]
            n199 = global read "总磷总氮断电保存全局变量.vi" "质控参数设置"() -> (w695:T9)
            n200 = case shown="\"标样核查\"" w709 {
              tunnel: w693 -> [w729 w736 w743 w750 w755 w760 w765]
              tunnel: [w728 w735 w742 w749 w754 w759 w764] -> w708
              tunnel: [w727 w734 w741 w748 w753 w758 w763] -> w707
              tunnel: [w726 w733 w740 w747 w752 w757 w762] -> w706
              tunnel: [T4."水样测试" ("测量模式") w730 T4."跨度核查" ("测量模式") T4."零点核查" ("测量模式") T4."加标回收" ("测量模式") w756 T4."平行样测试" ("测量模式")] -> w698
              tunnel: w695 -> [_ w732 w738 w745 _ _ _]
              tunnel: [_ w731 w737 w744 _ _ _] -> w705
              tunnel: w691 -> [_ _ _ _ _ w756 _]
              tunnel: w690 -> [_ w730 _ _ _ _ _]
              frame "水样测试", Default {
                n201 = Unbundle By Name(w729) -> ("水样数据时间"=w728:timestamp, "水样实测值"=w727:sgl, "水样数据标识"=w726:string)
              }
              frame "标样核查" {
                n202 = Unbundle By Name(w736) -> ("标样数据时间"=w735:timestamp, "标样实测值"=w734:sgl, "标样数据标识"=w733:string)
                n203 = Unbundle By Name(w732) -> ("COD标准液标准浓度"=w731:dbl)
              }
              frame "跨度核查" {
                n204 = Unbundle By Name(w743) -> ("跨度核查数据时间"=w742:timestamp, "跨度核查实测值"=w741:sgl, "跨度核查数据标识"=w740:string)
                n205 = Unbundle By Name(w738) -> ("COD跨度标准液浓度"=w737:dbl)
              }
              frame "零点核查" {
                n206 = Unbundle By Name(w750) -> ("零点核查数据时间"=w749:timestamp, "零点核查实测值"=w748:sgl, "零点核查数据标识"=w747:string)
                n207 = Unbundle By Name(w745) -> ("COD零点标准液浓度"=w744:dbl)
              }
              frame "加标回收" {
                n208 = Unbundle By Name(w755) -> ("加标回收数据时间"=w754:timestamp, "加标回收实测值"=w753:sgl, "加标回收数据标识"=w752:string)
              }
              frame "空白测试" {
                n209 = Unbundle By Name(w760) -> ("空白数据时间"=w759:timestamp, "空白实测值"=w758:sgl, "空白数据标识"=w757:string)
              }
              frame "平行样" {
                n210 = Unbundle By Name(w765) -> ("平行样数据时间"=w764:timestamp, "平行样实测值"=w763:sgl, "平行样数据标识"=w762:string)
              }
            }
            n211 = Unbundle By Name(w695) -> ("COD跨度值"=w694:dbl)
            n212 = And(x=w702, y=u16 255) -> (x .and. y?=w703:u16)
            n213 = case shown="0, 默认" w703 {
              tunnel: ["低量程" ("格式字符串") "高量程" ("格式字符串")] -> w701
              frame 0, Default {
              }
              frame 1 {
              }
            }
            n214 = global read "VAR总磷总氮全局变量.vi" "序列号"() -> (w700:string)
            n215 = Bundle By Name(cluster=w697, "时间标识"=w708, "监测值"=w707, "数据标识"=w706, "测量模式"=w698, "单位"=w722, "因子编码"=w721, "标样参考值"=w705, "F0"=w720, "F1"=w719, "F2"=w718, "F3"=w717, "F4"=w716, "F5"=w715, "F6"=w714, "F7"=w713, "X"=w712, "温度"=w711, "湿度"=w710, "量程标识"=w701, "SN"=w700, "数据标记表"=w699, "跨度值"=w694, "X1"=w688) -> (w696:T2)
            n216 = global read "VAR总磷总氮全局变量.vi" "CODcr关键参数"() -> (w689:T10)
            n217 = call "总磷氨氮插入数据.vi"("table"=w692, "关键参数"=w689, "data"=w696) -> ()  [unwired: 12 in, 1 out]
          }
        }
      }
    }
  }
